vi "getRfData.vi"(8 "error in (no error)":errorcluster, 11 "rf in":refnum<class "rf.lvclass">) -> (0 "error out":errorcluster, 2 "data":T1, 3 "rf out":refnum<class "rf.lvclass">)   [LabVIEW 2009, in "Tools.lvlib" / "Scripting.lvlib" / "rf.lvclass"]
uses:
  rf.lvclass
  DatabaseHelpers/Database Objects/Channel/RfOutputChannel/RfOutputChannel.lvclass
  rf.lvclass/rf.ctl
  ScriptEvent.lvclass
  xmlNode/xmlNode.lvclass
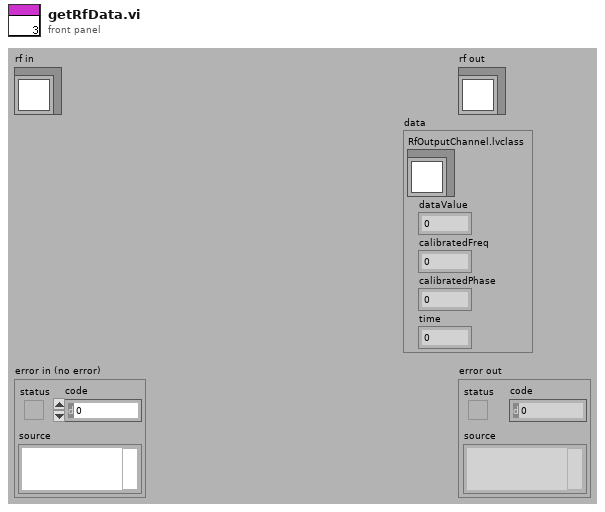
[diagram p1: front panel]
types:
  T1 = cluster{"RfOutputChannel.lvclass":refnum<class "RfOutputChannel.lvclass">, "dataValue":dbl, "calibratedFreq":dbl, "calibratedPhase":dbl, "time":dbl}
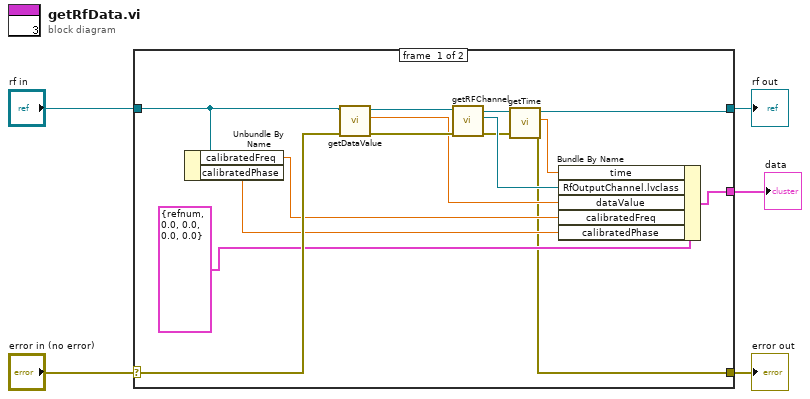
[diagram p0: block diagram]
diagram:
  n1 = case shown="No Error" "error in (no error)" {
    selector: "error in (no error)" -> [w19 w22]
    tunnel: [w7 w22] -> w4
    tunnel: [w6 w21] -> w2
    tunnel: "rf in" -> [w20 w21]
    tunnel: [w11 _] -> w1
    frame #0 {
      n2 = Unbundle By Name(w20) -> ("calibratedFreq"=w13:dbl, "calibratedPhase"=w12:dbl)
      n3 = call "getDataValue.vi"("error in (no error)"=w19, "ScriptEvent.lvclass in"=w20) -> ("error out"=w17:errorcluster, "dataValue"=w14:dbl, "ScriptEvent.lvclass out"=w18:refnum<class "rf.lvclass">)  [unwired: 7 in]
      n4 = call "getRFChannel.vi"("error in (no error)"=w17, "rf.lvclass in"=w18) -> ("error out"=w9:errorcluster, "RfOutputChannel.lvclass"=w15:refnum<class "RfOutputChannel.lvclass">, "rf.lvclass out"=w10:refnum<class "rf.lvclass">)  [unwired: 7 in]
      n5 = call "getTime.vi"("error in (no error)"=w9, "ScriptEvent.lvclass in"=w10) -> ("error out"=w7:errorcluster, "time"=w8:dbl, "ScriptEvent.lvclass out"=w6:refnum<class "rf.lvclass">)  [unwired: 7 in]
      n6 = Bundle By Name(cluster=T1 {"RfOutputChannel.lvclass"=refnum, "dataValue"=0.0, "calibratedFreq"=0.0, "calibratedPhase"=0.0, "time"=0.0} ("data"), "time"=w8, "RfOutputChannel.lvclass"=w15, "dataValue"=w14, "calibratedFreq"=w13, "calibratedPhase"=w12) -> (w11:T1)
    }
    frame #1 {
    }
  }
  "error out" <- w4
  "rf out" <- w2
  "data" <- w1
